vi "PRL Channel Names.vi"(6 "Details":T1, 7 "Initialize?":bool) -> (1 "Digital Signals":string[](array[string]), 2 "Analog Signals":string[](array[string]), 3 "Phasor Signals":string[](array[string]))   [LabVIEW 2013, in "PMU Recorder Light.lvlib"]
uses:
  PMU Recorder Light.lvlib
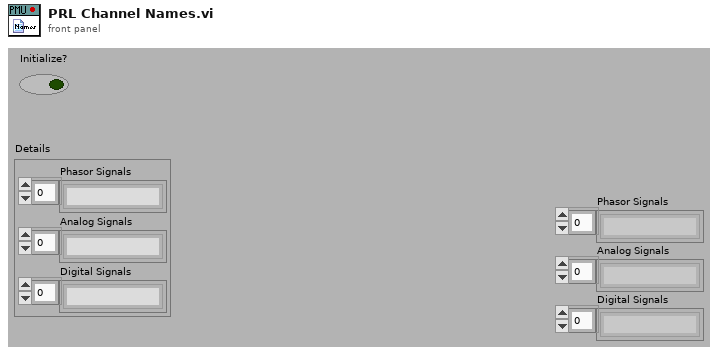
[diagram p1: front panel]
types:
  T1 = cluster{"Phasor Signals":string[], "Analog Signals":string[], "Digital Signals":string[]}
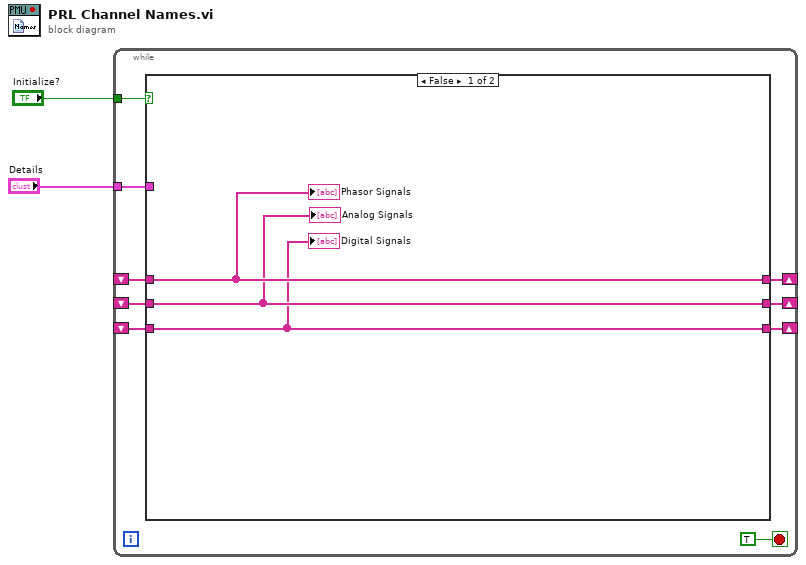
[diagram p0: block diagram]
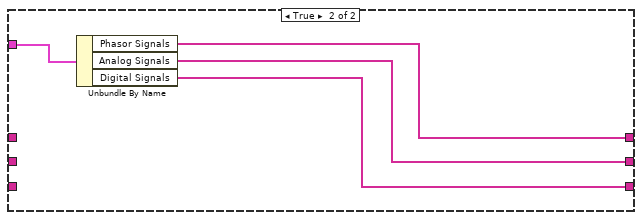
[diagram p2: hidden frame]
diagram:
  n1 = while {
    tunnel: "Initialize?" -> [w10]
    tunnel: "Details" -> [w9]
    shift-right: [w8] -> _
    shift-left: _ -> [w5]
    shift-right: [w7] -> _
    shift-left: _ -> [w4]
    shift-right: [w6] -> _
    shift-left: _ -> [w3]
    stop <- TRUE stop-if-true
    n2 = case shown="False" w10 {
      tunnel: w9 -> [_ w18]
      tunnel: [w14 w17] -> w8
      tunnel: [w13 w16] -> w7
      tunnel: [w12 w15] -> w6
      tunnel: w5 -> [w14 _]
      tunnel: w4 -> [w13 _]
      tunnel: w3 -> [w12 _]
      frame False {
        "Phasor Signals" <- w14
        "Analog Signals" <- w13
        "Digital Signals" <- w12
      }
      frame True {
        n3 = Unbundle By Name(w18) -> ("Phasor Signals"=w17:string[], "Analog Signals"=w16:string[], "Digital Signals"=w15:string[])
      }
    }
  }
